vi "get_section_key_value.vi"(10 "section_key_type_table":string[](array[string]), 11 "config_info":T1) -> (0 "type":string, 1 "value":string, 2 "key":string, 3 "section":string, 4 "index of element":i32)   [LabVIEW 2020]
uses:
  config_info.ctl
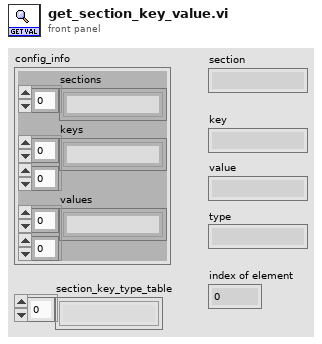
[diagram p1: front panel]
types:
  T1 = typedef "config_info.ctl" = cluster{"sections":string[], "keys":string[][], "values":string[][]}
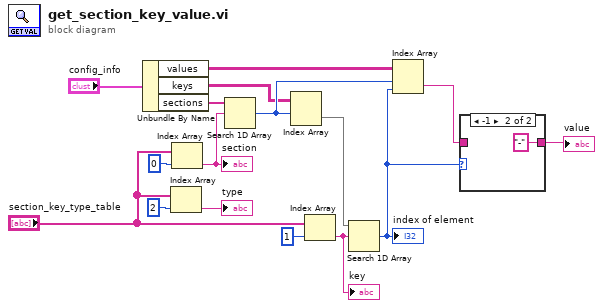
[diagram p0: block diagram]
diagram:
  n1 = Unbundle By Name("config_info") -> ("values"=w10:string[][], "keys"=w7:string[][], "sections"=w6:string[])
  n2 = Index Array(array="section_key_type_table", index=2) -> (element=→"type":string)
  n3 = Index Array(array="section_key_type_table", index=0) -> (element=w16:string)
  "section" <- w16
  n4 = Search 1D Array(1D array=w6, element=w16) -> (index of element=w11:i32)  [unwired: 1 in]
  n5 = Index Array(array=w7, index (row)=w11) -> (element=w8:string[])  [unwired: 1 in]
  n6 = Index Array(array="section_key_type_table", index=1) -> (element=w15:string)
  "key" <- w15
  n7 = Search 1D Array(1D array=w8, element=w15) -> (index of element=w3:i32)  [unwired: 1 in]
  "index of element" <- w3
  n8 = Index Array(array=w10, index (row)=w11, index (col)=w3) -> (element=w2:string)
  n9 = case shown="-1" w3 {
    tunnel: w2 -> [w17 _]
    tunnel: [w17 "-" ("value")] -> w1
    frame Default {
    }
    frame -1 {
    }
  }
  "value" <- w1
